vi "Pre Launch Init.vi"(11 "IED Test in":refnum<class "IED Test.lvclass">) -> (0 "error out":errorcluster, 3 "IED Test out":refnum<class "IED Test.lvclass">)   [LabVIEW 2018, in "IED Test Framework.lvlib" / "IED Test.lvclass"]
doc: "(<B>Filename</B>: Actor Framework.lvlib:Actor.lvclass:Pre Launch Init.vi)\n\nDefines behavior that occurs after the Launch Nested Actor method is invoked but before the actor's Actor Core method begins running.\n\nBy default, this method does nothing. A descendant class may override it to define behavior."
uses:
  IED Test.lvclass
  C:/Users/Administrator/Desktop/2018LabVIEW EMS/EMS Generic Actor/EMS Generic/EMS Generic.lvclass
  EMS Generic Actor/EMS Generic/EMS Generic.lvclass/EMS Generic.ctl
  EMS Generic Actor/EMS Generic/EMS Generic.lvclass
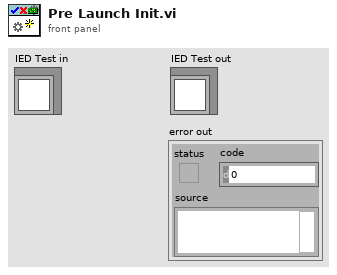
[diagram p1: front panel]
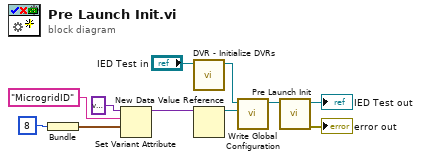
[diagram p0: block diagram]
diagram:
  n1 = Bundle("MicrogridID"=u8 8) -> (w8:cluster{"MicrogridID":u8})  [unwired: 1 in]
  n2 = Set Variant Attribute(Variant=variant ("variant"), name="MicrogridID", value=w8) -> (Variant out=w6:variant)  [unwired: 1 in, 2 out]
  n3 = call "DVR - Initialize DVRs.vi"("EMS Generic in"="IED Test in") -> ("EMS Generic out"=w2:refnum<class "IED Test.lvclass">)  [unwired: 9 in, 1 out]
  n4 = New Data Value Reference(data value=w6) -> (data value reference=w7:refnum<data-value>)  [unwired: 1 in, 1 out]
  n5 = call "Write Global Configuration.vi"("Global Configuration"=w7, "EMS Generic in"=w2) -> ("EMS Generic out"=w1:refnum<class "IED Test.lvclass">)  [unwired: 9 in]
  n6 = call-parent "Pre Launch Init.vi"("EMS Generic in"=w1) -> ("error out"=→"error out":errorcluster, "EMS Generic out"=→"IED Test out":refnum<class "IED Test.lvclass">)  [unwired: 9 in]
